vi "img.saveIndividual.vi"(5 "vars":T1={"save"={"base_folder"={"Folder"=path "", "tif"=FALSE, "jpg"=FALSE}, "module"="", "#"=20, "sub#"=0, "save.op"=enum."Full", "same?"=FALSE, "Shift"=enum."Single", "jpg?"=FALSE, "flip"={"x"=FALSE, "y"=FALSE}}, "acq"={"# Acq"=100, "rotate"=FALSE}, "calib.manual"={"BG"={"Image"=[], "enabled?"=FALSE}, "FF"={"Image"=[], "enabled?"=FALSE}}}, 6 "loop":i32, 7 "path":path, 8 "error in":errorcluster, 9 "Dark":u16[][](array[numeric]), 10 "PL":u16[][](array[numeric]), 11 "Bright":u16[][](array[numeric])) -> (0 "error out":errorcluster)   [LabVIEW 2020]
uses:
  _controls/data.vars.ctl
  _controls/flip.ctl
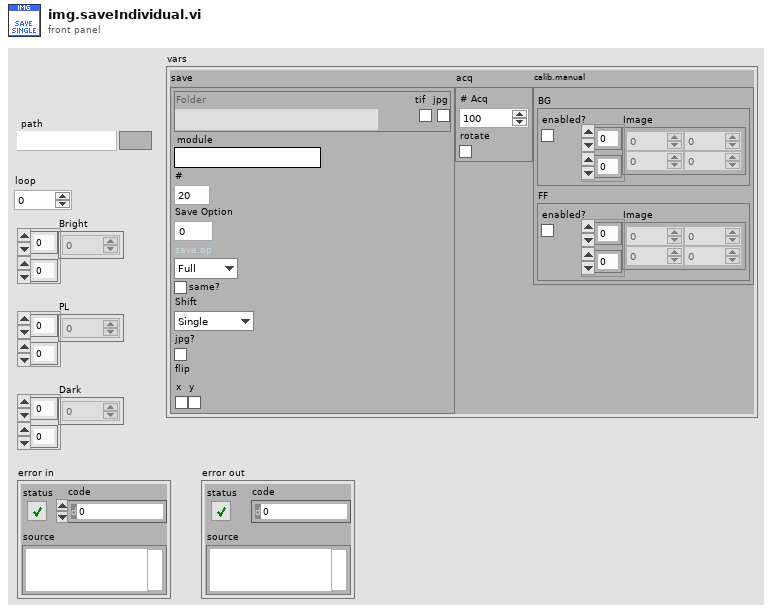
[diagram p1: front panel]
types:
  T1 = typedef "data.vars.ctl" = cluster{"save":cluster{"base_folder":cluster{"Folder":path, "tif":bool, "jpg":bool}, "module":string, "#":u32, "sub#":u8, "save.op":enum16{"Full", "Light"}, "same?":bool, "Shift":enum16{"Single", "Leapfrog"}, "jpg?":bool, "flip":T2}, "acq":cluster{"# Acq":u16, "rotate":bool}, "calib.manual":cluster{"BG":cluster{"Image":u16[][], "enabled?":bool}, "FF":cluster{"Image":u16[][], "enabled?":bool}}}
  T2 = typedef "flip.ctl" = cluster{"x":bool, "y":bool}
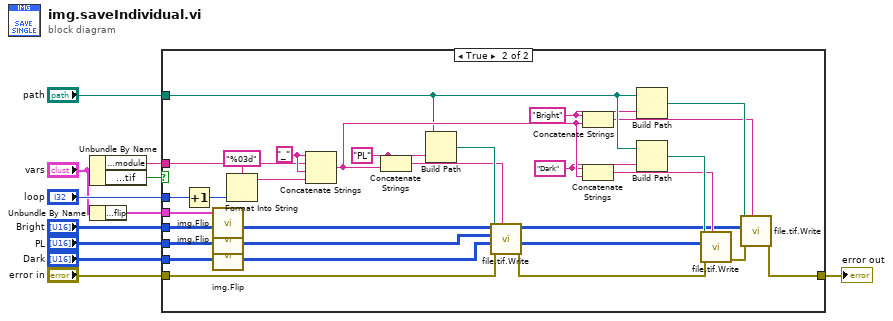
[diagram p0: block diagram]
diagram:
  n1 = Unbundle By Name("vars") -> ("save.module"=w4:string, "save.base_folder.tif"=w3:bool)
  n2 = Unbundle By Name("vars") -> ("save.flip"=w1:T2)
  n3 = case shown="True" w3 {
    tunnel: "Dark" -> [_ w18]
    tunnel: "PL" -> [_ w17]
    tunnel: "Bright" -> [_ w19]
    tunnel: "error in" -> [w12 w40]
    tunnel: "path" -> [_ w33]
    tunnel: [w12 w32] -> w6
    tunnel: "loop" -> [_ w28]
    tunnel: w4 -> [_ w27]
    tunnel: w1 -> [_ w14]
    frame False {
    }
    frame True {
      w30 = "Dark" ("String")
      w29 = "Bright" ("String")
      w39 = "PL" ("String")
      w34 = "_" ("string")
      n4 = Increment(x=w28) -> (x+1=w38:i32)
      n5 = call "img.Flip.vi"("flip"=w14, "image in"=w19) -> ("image out"=w16:u16[][])  [unwired: 9 in]
      n6 = call "img.Flip.vi"("flip"=w14, "image in"=w17) -> ("image out"=w15:u16[][])  [unwired: 9 in]
      n7 = call "img.Flip.vi"("flip"=w14, "image in"=w18) -> ("image out"=w13:u16[][])  [unwired: 9 in]
      n8 = Format Into String(format string="%03d", w38) -> (resulting string=w36:string)  [unwired: 2 in, 1 out]
      n9 = Concatenate Strings(w34, w27, w34, w36) -> (w35:string)
      n10 = Concatenate Strings(w39, w35) -> (w21:string)
      n11 = Build Path(base path=w33, name or relative path=w39) -> (appended path=w22:path)
      n12 = call "file.tif.Write.vi"("name"=w21, "error in"=w40, "u16 pixmap"=w15, "path"=w22) -> ("error out"=w31:errorcluster)  [unwired: 7 in]
      n13 = Concatenate Strings(w29, w35) -> (w24:string)
      n14 = Concatenate Strings(w30, w35) -> (w23:string)
      n15 = Build Path(base path=w33, name or relative path=w29) -> (appended path=w25:path)
      n16 = Build Path(base path=w33, name or relative path=w30) -> (appended path=w26:path)
      n17 = call "file.tif.Write.vi"("name"=w23, "error in"=w31, "u16 pixmap"=w13, "path"=w26) -> ("error out"=w20:errorcluster)  [unwired: 7 in]
      n18 = call "file.tif.Write.vi"("name"=w24, "error in"=w20, "u16 pixmap"=w16, "path"=w25) -> ("error out"=w32:errorcluster)  [unwired: 7 in]
    }
  }
  "error out" <- w6
